vi "RSNRPZ Get Statistics Scale Ref Level.vi"(8 "error in (no error)":errorcluster, 10 "Channel (1)":i32=1, 11 "VISA session":refnum<visa-resource-name> caption="VISA resource name") -> (0 "error out":errorcluster, 2 "Reference Level":dbl format="%^.3e", 3 "dup VISA session":refnum<visa-resource-name> caption="VISA resource name")   [LabVIEW 2010]
doc: "This VI queries the lower limit of the level range for the analysis result in both Statistics modes. This level can be assigned to the first pixel. The level assigned to the last pixel is equal to the level of the first pixel plus the level range.\n\nRemote-control command(s):\nSENSe:STATistics:SCALE:X:RLEVel?"
uses:
  rsnrpz_32.dll
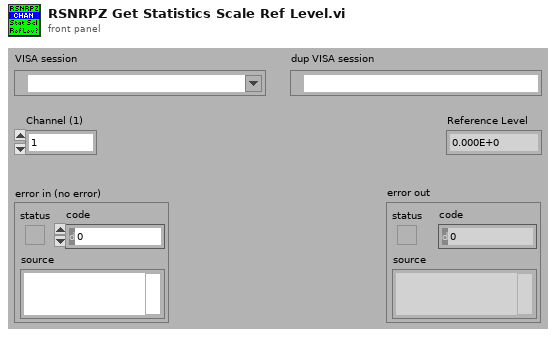
[diagram p1: front panel]
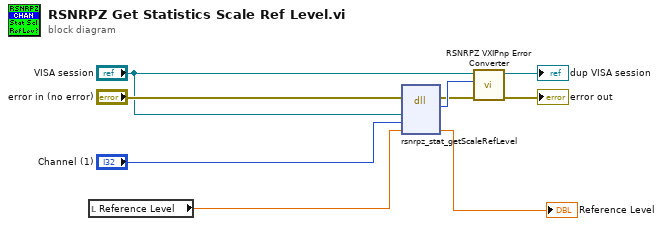
[diagram p0: block diagram]
diagram:
  n1 = local read "Reference Level"() -> (w7:dbl)
  n2 = dll-call lib="rsnrpz_32.dll" fn="rsnrpz_stat_getScaleRefLevel"(error in="error in (no error)", "Instrument Handle"="VISA session", "Channel"="Channel (1)", "Reference Level"=w7) -> (error out=w5:errorcluster, "Status"=w9:i32, "Reference Level"=→"Reference Level":dbl)  [unwired: 4 in, 1 out]
  n3 = call <instrlib>:"RSNRPZ VXIPnp Error Converter.vi"("error in"=w5, "VXIPnp error code"=w9, "VISA session"="VISA session") -> ("error out"=→"error out":errorcluster, "dup VISA session"=→"dup VISA session":refnum<visa-resource-name>)  [unwired: 7 in]
